vi "Format Subpage Link.vi"(8 "error in (no error)":errorcluster {"code" format="Error %.0f"}, 10 "Qualified Name":string, 11 "VIDoc Printer - Confluence In":refnum<class "VIDoc Printer - Confluence.lvclass">) -> (0 "error out":errorcluster {"code" format="Error %.0f"}, 2 "Linked HTML":string, 3 "VIDoc Printer - Confluence Out":refnum<class "VIDoc Printer - Confluence.lvclass">)   [LabVIEW 2023, in "VIDoc Printer - Confluence.lvlib" / "VIDoc Printer - Confluence.lvclass"]
uses:
  VIDoc Printer - Confluence.lvclass
  VIDoc Printer - Confluence.lvclass/VIDoc Printer - Confluence.ctl
  <userlib>/_PetranWay/LabVIEW Confluence API/Source/Confluence/HTML/Add Link to Text/Add Anchor To Text.vi
  <userlib>/_PetranWay/LabVIEW Confluence API/Source/PetranWay_Confluence API.lvlib
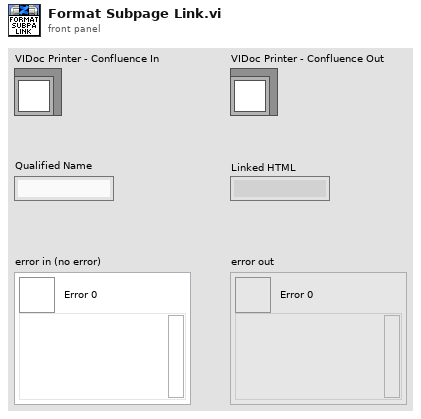
[diagram p1: front panel]
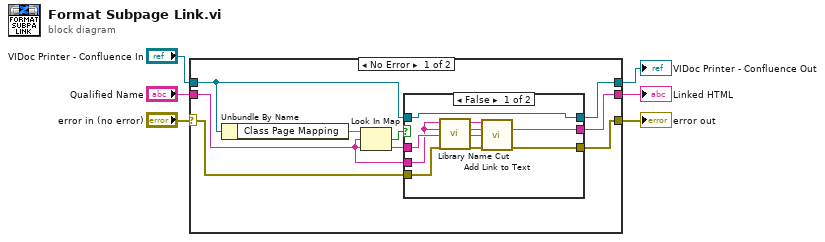
[diagram p0: block diagram]
diagram:
  n1 = case shown="No Error" "error in (no error)" {
    selector: "error in (no error)" -> [w14 w27]
    tunnel: [w13 w27] -> w5
    tunnel: [w15 w26] -> w3
    tunnel: "VIDoc Printer - Confluence In" -> [w11 w26]
    tunnel: [w12 _] -> w2
    tunnel: "Qualified Name" -> [w8 _]
    frame No Error {
      n2 = Unbundle By Name(w11) -> ("Class Page Mapping"=w10:map{string, string})
      n3 = Look In Map(map=w10, key=w8, default value=w8) -> (key not found?=w7:bool, value=w9:string)
      n4 = case shown="False" w7 {
        tunnel: [w22 w25] -> w15
        tunnel: w14 -> [w21 w23]
        tunnel: [w20 w23] -> w13
        tunnel: [w19 w24] -> w12
        tunnel: w11 -> [w22 w25]
        tunnel: w9 -> [w18 _]
        tunnel: w8 -> [w17 w24]
        frame False {
          n5 = call "Library Name Cut.vi"("Name in"=w17) -> ("Name out"=w16:string)  [unwired: 10 in]
          n6 = call-poly <userlib>:"Add Link to Text.vi"("Link Text"=w16, "Anchor Name"=w17, "Page Name"=w18, "error in (no error)"=w21) -> ("Anchor HTML"=w19:string, "error out"=w20:errorcluster)  [unwired: 9 in, 1 out]
        }
        frame True {
        }
      }
    }
    frame Error {
    }
  }
  "error out" <- w5
  "VIDoc Printer - Confluence Out" <- w3
  "Linked HTML" <- w2
